vi "Edit VI String Constant.vi"(7 "string label":string="CD Name", 8 "error in":errorcluster, 9 "new value":string, 10 "relative path of VI to edit":path, 11 "custom device path":path) -> (0 "error out":errorcluster, 3 "custom device path out":path)   [LabVIEW 2020, in "Template Tool.lvlib"]
uses:
  Template Tool.lvlib
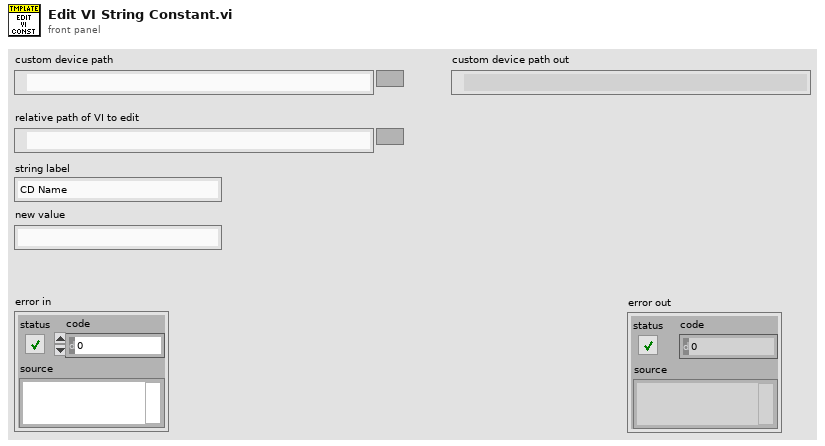
[diagram p1: front panel]
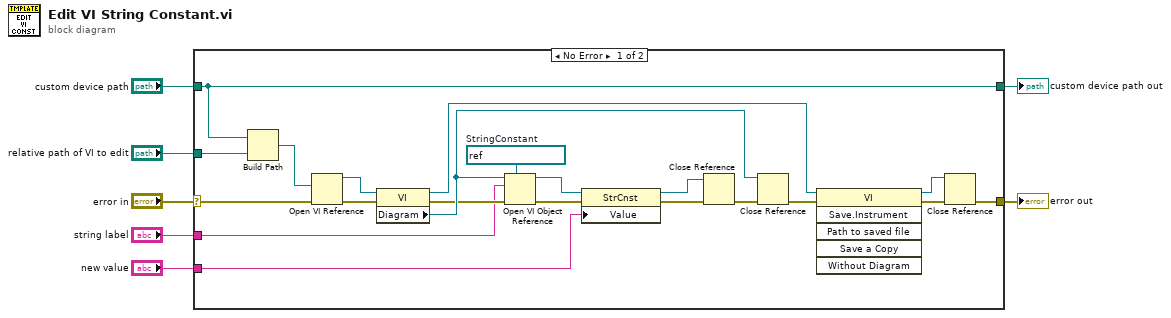
[diagram p0: block diagram]
diagram:
  n1 = case shown="No Error" "error in" {
    selector: "error in" -> [w22 w29]
    tunnel: [w15 w29] -> w7
    tunnel: "custom device path" -> [w23 w30]
    tunnel: "relative path of VI to edit" -> [w24 _]
    tunnel: [w23 w30] -> w4
    tunnel: "new value" -> [w9 _]
    tunnel: "string label" -> [w8 _]
    frame No Error {
      w13 = refnum<vi> refnum  # StringConstant
      n2 = Build Path(base path=w23, name or relative path=w24) -> (appended path=w26:path)
      n3 = Open VI Reference(vi path=w26, error in (no error)=w22) -> (vi reference=w27:refnum<vi>, error out=w28:errorcluster)  [unwired: 4 in]
      n4 = property class="VI"(reference=w27, error in=w28) -> (reference out=w25:refnum<vi>, error out=w14:errorcluster, "Diagram"=w20:refnum<vi>)
      n5 = Open VI Object Reference(7:w13, 8:w14, 10:w8, 11:w20) -> (0:w12:errorcluster, 3:w11:refnum<vi>)
      n6 = property class="StrCnst"(reference=w11, error in=w12, "Value"=w9) -> (reference out=w10:refnum<vi>, error out=w19:errorcluster)
      n7 = Close Reference(reference=w10, error in (no error)=w19) -> (error out=w21:errorcluster)
      n8 = Close Reference(reference=w20, error in (no error)=w21) -> (error out=w18:errorcluster)
      n9 = invoke class="VI" method="Save.Instrument"(reference=w25, error in=w18) -> (reference out=w17:refnum<vi>, error out=w16:errorcluster)  [unwired: 4 in, 4 out]
      n10 = Close Reference(reference=w17, error in (no error)=w16) -> (error out=w15:errorcluster)
    }
    frame Error {
    }
  }
  "error out" <- w7
  "custom device path out" <- w4
